vi "DAC Configure.vi"(8 "error in":errorcluster, 11 "DAC HeatFlow Load dU in":refnum<class "DAC HeatFlow Load dU.lvclass">) -> (0 "error out":errorcluster, 3 "DAC HeatFlow Load dU out":refnum<class "DAC HeatFlow Load dU.lvclass">)   [LabVIEW 2019, in "DAC.lvlib" / "DAC HeatFlow Load dU.lvclass"]
uses:
  DAC HeatFlow Load dU.lvclass
  C:/Users/krio/Documents/LV_Projects/test-stand/App/DAC/DAC.lvclass
  DAC.lvclass/DAC.ctl
  DAC HeatFlow Load dU.lvclass/DAC HeatFlow Load dU.ctl
  <vilib>/Utility/error.llb/Error Cluster From Error Code.vi
  <vilib>/DAQmx/create/channels.llb/DAQmx Create Channel (AI-Voltage-Basic).vi
  <vilib>/ErrorRing/Error Ring.xnode
  DAC.lvclass
  <resource>/objmgr/daqmx.rc
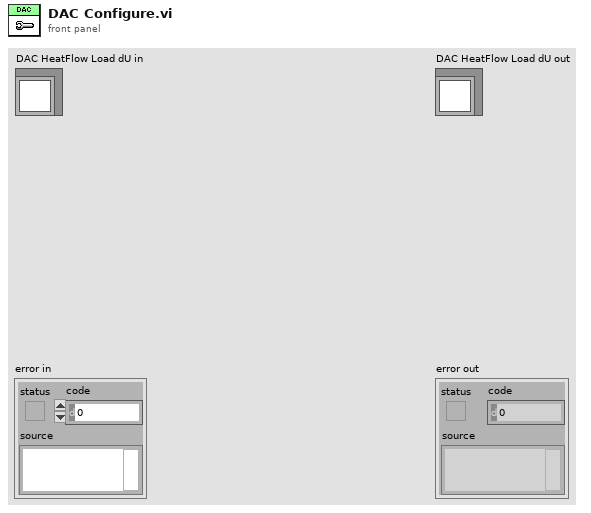
[diagram p1: front panel]
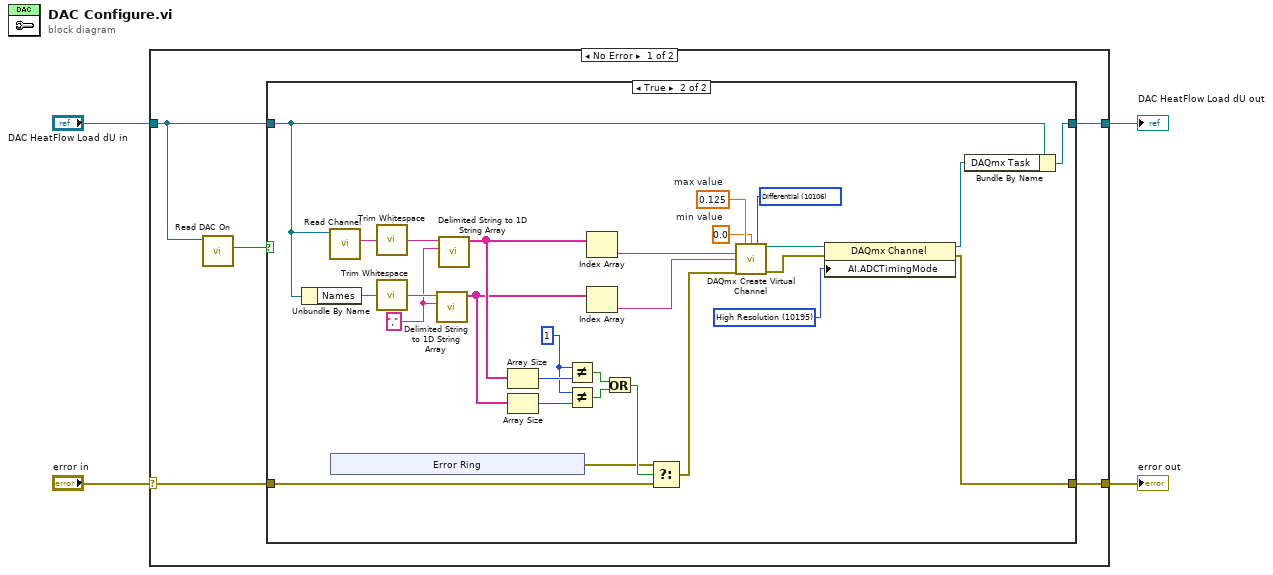
[diagram p0: block diagram]
diagram:
  n1 = case shown="No Error" "error in" {
    selector: "error in" -> [w6 w45]
    tunnel: [w5 w45] -> w4
    tunnel: [w7 w44] -> w3
    tunnel: "DAC HeatFlow Load dU in" -> [w9 w44]
    frame No Error {
      n2 = call "Read DAC On.vi"("DAC in"=w9) -> ("DAC On"=w8:bool)  [unwired: 8 in, 2 out]
      n3 = case shown="True" w8 {
        tunnel: w9 -> [w11 w38]
        tunnel: [w11 w39] -> w7
        tunnel: w6 -> [w10 w23]
        tunnel: [w10 w12] -> w5
        frame False {
        }
        frame True {
          w14 = 10195 items=["Automatic"=16097, "High Resolution"=10195, "High Speed"=14712, "Best 50 Hz Rejection"=14713, "Best 60 Hz Rejection"=14714, "Custom"=10137] ("AI.ADCTimingMode")
          w27 = 1 ("x")
          w30 = "," ("delimiter")
          w35 = 10106 items=["Default"=-1, "RSE"=10083, "NRSE"=10078, "Differential"=10106, "Pseudodifferential"=12529] ("input terminal configuration")
          w36 = 0.0  # min value
          w37 = 0.125  # max value
          n4 = Unbundle By Name(w38) -> ("Names"=w33:string)
          n5 = call "Read Channel.vi"("DAC in"=w38) -> ("Channel"=w34:string)  [unwired: 8 in, 2 out]
          n6 = xnode "Error Ring"() -> ("error out"=w22:errorcluster)
          n7 = call <vilib>:"Trim Whitespace.vi"("string"=w34) -> ("trimmed string"=w32:string)  [unwired: 1 in]
          n8 = call <vilib>:"Trim Whitespace.vi"("string"=w33) -> ("trimmed string"=w31:string)  [unwired: 1 in]
          n9 = call <vilib>:"Delimited String to 1D String Array.vi"("delimiter"=w30, "delimited string"=w31) -> ("string array"=w20:string[])  [unwired: 9 in]
          n10 = call <vilib>:"Delimited String to 1D String Array.vi"("delimiter"=w30, "delimited string"=w32) -> ("string array"=w21:string[])  [unwired: 9 in]
          n11 = Array Size(array=w21) -> (size(s)=w29:i32)
          n12 = Array Size(array=w20) -> (size(s)=w28:i32)
          n13 = Not Equal?(x=w27, y=w29) -> (x != y?=w26:bool)
          n14 = Not Equal?(x=w27, y=w28) -> (x != y?=w25:bool)
          n15 = Index Array(array=w21) -> (element=w19:string)  [unwired: 1 in]
          n16 = Index Array(array=w20) -> (element=w18:string)  [unwired: 1 in]
          n17 = Or(x=w26, y=w25) -> (x .or. y?=w24:bool)
          n18 = Select(t=w22, s=w24, f=w23) -> (s? t:f=w17:errorcluster)
          n19 = call-poly <vilib>:"DAQmx Create Virtual Channel.vi"("maximum value"=w37, "minimum value"=w36, "input terminal configuration"=w35, "physical channels"=w19, "name to assign"=w18, "error in"=w17) -> ("task out"=w16:refnum<k21>, "error out"=w15:errorcluster)  [unwired: 8 in]
          n20 = property class="DAQmx Channel"(reference=w16, error in=w15, "AI.ADCTimingMode"=w14) -> (reference out=w13:refnum<k21>, error out=w12:errorcluster)
          n21 = Bundle By Name(cluster=w38, "DAQmx Task"=w13) -> (w39:refnum<class "DAC HeatFlow Load dU.lvclass">)
        }
      }
    }
    frame Error {
    }
  }
  "error out" <- w4
  "DAC HeatFlow Load dU out" <- w3
